vi "Read List Steps.vi"(8 "error in (no error)":errorcluster, 11 "VISA resource name":refnum<visa-resource-name>) -> (0 "error out":errorcluster, 2 "List Step Count":dbl, 3 "VISA resource name out":refnum<visa-resource-name>)   [LabVIEW 2015, in "IT6700H.lvlib"]
doc: "Gets the total number of steps in the list."
uses:
  <instrlib>/IT6700H/IT6700H.lvlib
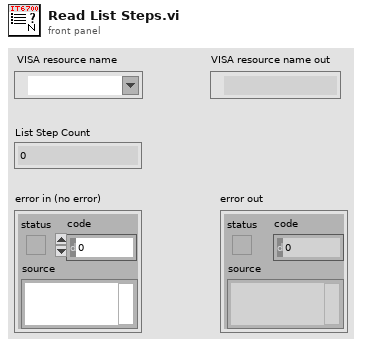
[diagram p1: front panel]
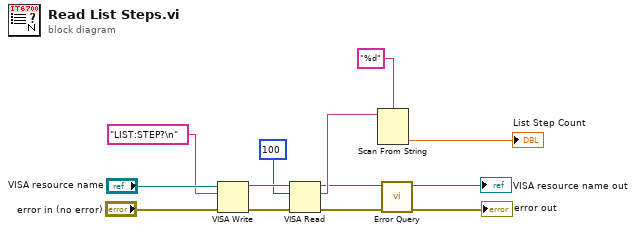
[diagram p0: block diagram]
diagram:
  n1 = VISA Write(VISA resource name="VISA resource name", write buffer="LIST:STEP?\n", error in (no error)="error in (no error)") -> (VISA resource name out=w9:refnum<visa-resource-name>, error out=w10:errorcluster)  [unwired: 1 out]
  n2 = VISA Read(VISA resource name=w9, byte count=100, error in (no error)=w10) -> (VISA resource name out=w5:refnum<visa-resource-name>, read buffer=w7:string, error out=w6:errorcluster)  [unwired: 1 out]
  n3 = Scan From String(format string="%d", input string=w7) -> (output 1=→"List Step Count":dbl)  [unwired: 3 in, 3 out]
  n4 = call <instrlib>:"Error Query.vi"("error in (no error)"=w6, "VISA resource name"=w5) -> ("error out"=→"error out":errorcluster, "VISA resource name out"=→"VISA resource name out":refnum<visa-resource-name>)  [unwired: 6 in, 2 out]
